vi "TakeReading.vi"(8 "error in":errorcluster, 11 "Port":refnum<visa-resource-name>) -> (0 "error out":errorcluster, 1 "Frequency":dbl, 2 "Voltage(mV)":dbl, 3 "Port out":refnum<visa-resource-name>)   [LabVIEW 2018]
uses:
  <vilib>/Instr/_visa.llb/VISA Flush IO Buffer Mask.ctl
panel:
  out "read buffer":string
  out "Value":dbl
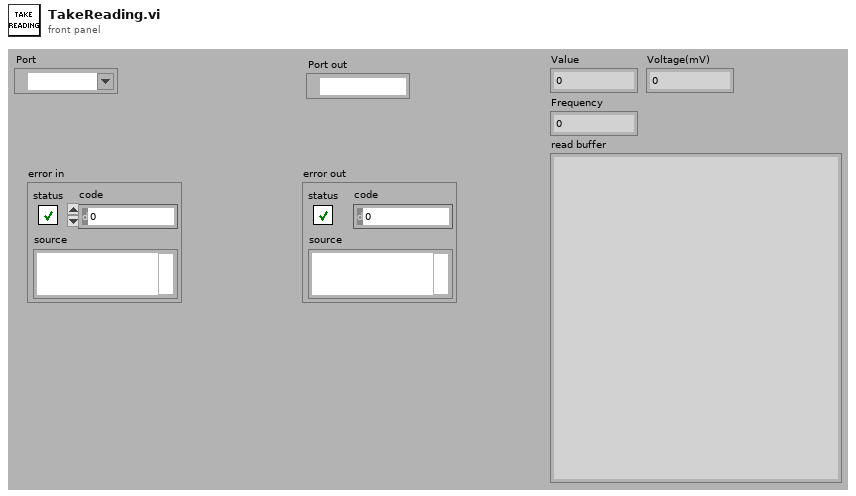
[diagram p1: front panel]
types:
  T1 = typedef "VISA Flush IO Buffer Mask.ctl" = u16
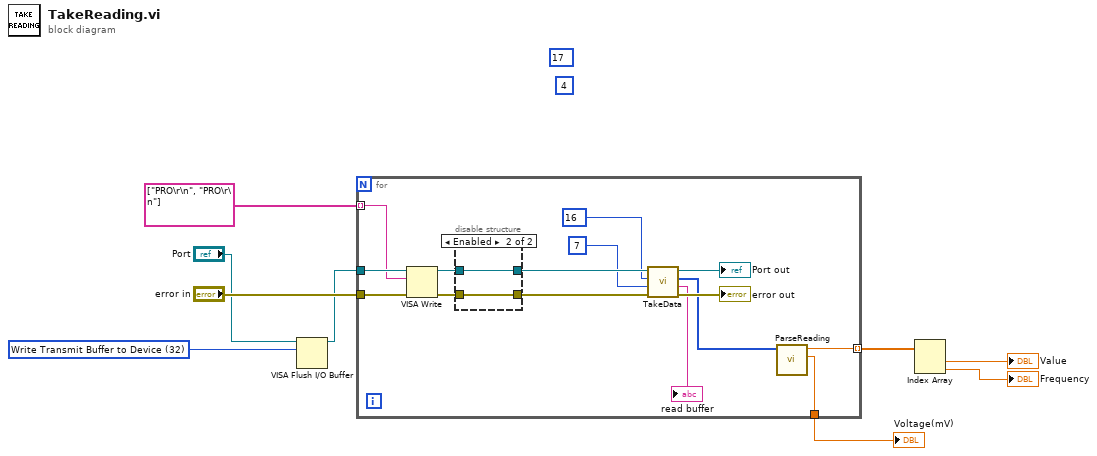
[diagram p0: block diagram]
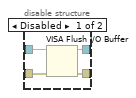
[diagram p2: hidden frame]
diagram:
  (unwired) u32 17 ("Location")
  (unwired) u32 4 ("Location")
  w4 = T1 32 items=["Flush Receive Buffer"=16, "Write Transmit Buffer to Device"=32, "Flush Receive Buffer (No I/O)"=64, "Flush Transmit Buffer"=128] ("Mask")
  n1 = VISA Flush I/O Buffer(VISA resource name="Port", mask (16)=w4) -> (VISA resource name out=w2:refnum<visa-resource-name>)  [unwired: 1 in, 1 out]
  n2 = for {
    tunnel: [w23] -> w7 mode=indexing
    tunnel: w2 -> [w22]
    tunnel: "error in" -> [w21]
    tunnel: string[] ["PRO\r\n", "PRO\r\n"] ("concatenated string") -> [w20] mode=indexing
    tunnel: [w10] -> w1
    n3 = VISA Write(VISA resource name=w22, write buffer=w20, error in (no error)=w21) -> (VISA resource name out=w17:refnum<visa-resource-name>, error out=w16:errorcluster)  [unwired: 1 out]
    n4 = disable-structure shown="Enabled" {
      disable-tunnel: w17 -> [w28 w30]
      disable-tunnel: w16 -> [w27 w29]
      disable-tunnel: [w26 w29] -> w15
      disable-tunnel: [w25 w30] -> w14
      frame Disabled {
        n5 = VISA Flush I/O Buffer(VISA resource name=w28, error in (no error)=w27) -> (VISA resource name out=w25:refnum<visa-resource-name>, error out=w26:errorcluster)  [unwired: 1 in]
      }
      frame Enabled {
      }
    }
    n6 = call "TakeData.vi"("error in"=w15, "#words"=u32 7 ("Location"), "Location"=u32 16, "Port"=w14) -> ("error out"=→"error out":errorcluster, "read buffer"=→"read buffer":string, "Data"=w19:u16[], "Port out"=→"Port out":refnum<visa-resource-name>)  [unwired: 4 in]
    n7 = call "ParseReading.vi"("Data"=w19) -> ("Voltage"=w10:dbl, "Freq"=w23:dbl)  [unwired: 9 in]
  }
  "Voltage(mV)" <- w1
  n8 = Index Array(array=w7) -> (element #1=→"Value":dbl, element #2=→"Frequency":dbl)  [unwired: 2 in]
